vi "popCommand.vi"(8 "error in (no error)":errorcluster, 11 "CommandQueue in":refnum<class "CommandQueue.lvclass">) -> (0 "error out":errorcluster, 2 "Command":refnum<class "Command.lvclass">, 3 "CommandQueue out":refnum<class "CommandQueue.lvclass">)   [LabVIEW 2020, in "CommandQueue.lvclass"]
uses:
  CommandQueue.lvclass
  Command/Command.lvclass
  CommandQueue.lvclass/CommandQueue.ctl
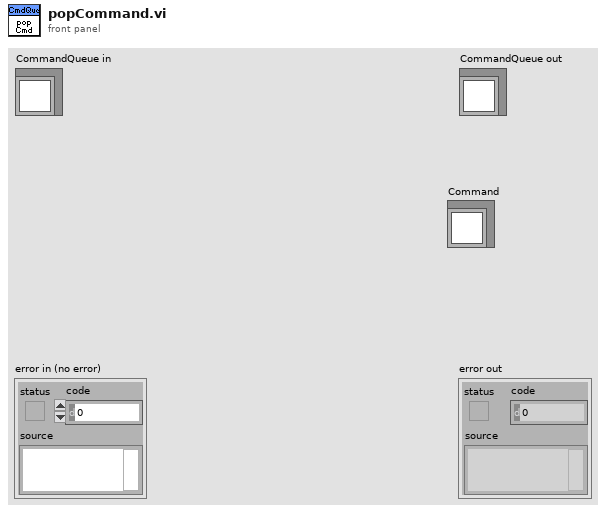
[diagram p1: front panel]
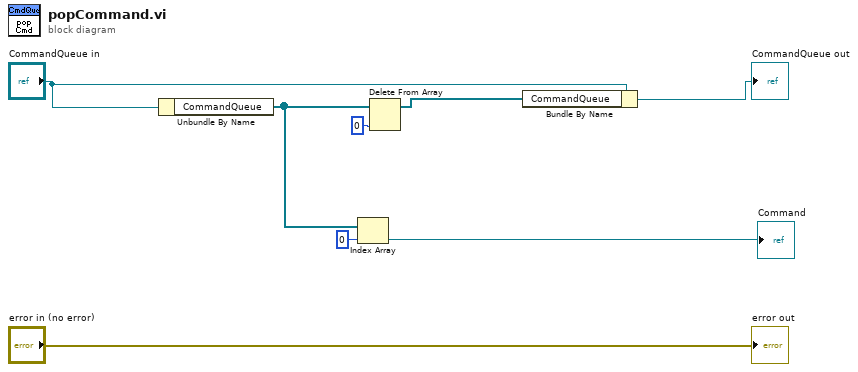
[diagram p0: block diagram]
diagram:
  n1 = Unbundle By Name("CommandQueue in") -> ("CommandQueue"=w3:refnum<class "Command.lvclass">[])
  n2 = Index Array(array=w3, index=0) -> (element=→"Command":refnum<class "Command.lvclass">)
  n3 = Delete From Array(array=w3, index=0) -> (array with subset deleted=w1:refnum<class "Command.lvclass">[])  [unwired: 1 in, 1 out]
  n4 = Bundle By Name(cluster="CommandQueue in", "CommandQueue"=w1) -> (→"CommandQueue out":refnum<class "CommandQueue.lvclass">)
  "error out" <- "error in (no error)"
